vi "Generate Configuration.vi"(6 "Starting Address Offset":u16 format="%04x", 7 "Virtual Memory Unit in":refnum<class "Virtual Memory Unit.lvclass">, 8 "error in (no error)":errorcluster, 11 "Bus Controller in":refnum<class "Bus Controller.lvclass">) -> (0 "error out":errorcluster, 2 "Parameter List":string[](array[string]), 3 "Bus Controller out":refnum<class "Bus Controller.lvclass">, 4 "Next Address Offset":u16 format="%04x", 5 "Virtual Memory Unit out":refnum<class "Virtual Memory Unit.lvclass">)   [LabVIEW 2020, in "BCI-1553 API.lvlib" / "Bus Controller.lvclass"]
doc: "Generates the entire configuration for this Bus Controller. Does not push it to the Board component yet."
uses:
  Bus Controller.lvclass
  C:/Users/MattJ/Desktop/git/bci-1553-labview-api/src/1553 SubComponent/1553 SubComponent.lvclass
  Dependencies/Virtual Memory Unit/Virtual Memory Unit.lvclass
  Dependencies/Registry/Registry.lvclass/Registry.ctl
  Dependencies/Registry/Registry.lvclass
  1553 SubComponent/1553 SubComponent.lvclass
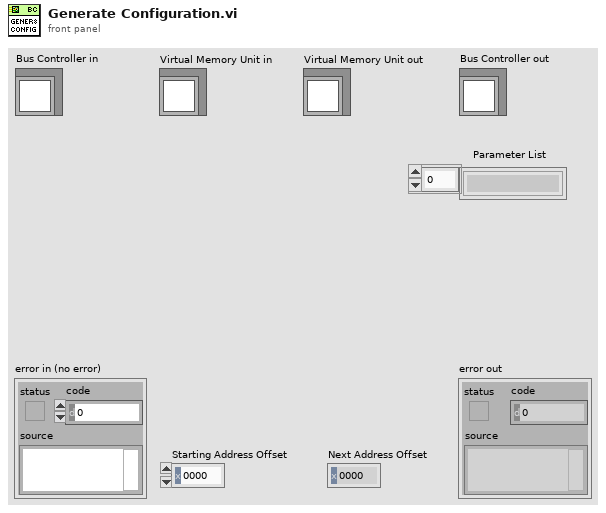
[diagram p1: front panel]
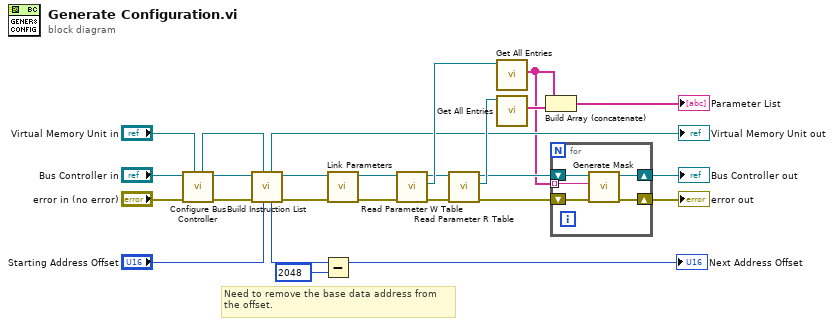
[diagram p0: block diagram]
diagram:
  # "Need to remove the base data address from\nthe offset."
  n1 = call "Configure Bus Controller.vi"("Virtual Memory Unit in"="Virtual Memory Unit in", "error in (no error)"="error in (no error)", "Bus Controller in"="Bus Controller in") -> ("error out"=w18:errorcluster, "Bus Controller out"=w21:refnum<class "Bus Controller.lvclass">, "Virtual Memory Unit out"=w14:refnum<class "Virtual Memory Unit.lvclass">)  [unwired: 6 in]
  n2 = call "Build Instruction List.vi"("Instruction List Starting Offset"="Starting Address Offset", "Virtual Memory Unit in"=w14, "error in (no error)"=w18, "Bus Controller in"=w21) -> ("error out"=w11:errorcluster, "Bus Controller out"=w12:refnum<class "Bus Controller.lvclass">, "Instruction List Final Address"=w3:u16, "Virtual Memory Unit out"=→"Virtual Memory Unit out":refnum<class "Virtual Memory Unit.lvclass">)  [unwired: 4 in]
  n3 = Subtract(x=w3, y=u16 2048) -> (x-y=→"Next Address Offset":u16)
  n4 = call "Link Parameters.vi"("error in (no error)"=w11, "Bus Controller in"=w12) -> ("error out"=w16:errorcluster, "Bus Controller out"=w19:refnum<class "Bus Controller.lvclass">)  [unwired: 8 in]
  n5 = call-dynamic "Read Parameter W Table.vi"("error in (no error)"=w16, "1553 SubComponent in"=w19) -> ("error out"=w26:errorcluster, "Parameter W Table"=w25:refnum<class "Registry.lvclass">, "1553 SubComponent out"=w23:refnum<class "Bus Controller.lvclass">)  [unwired: 7 in]
  n6 = call-dynamic "Read Parameter R Table.vi"("error in (no error)"=w26, "1553 SubComponent in"=w23) -> ("error out"=w8:errorcluster, "Parameter R Table"=w24:refnum<class "Registry.lvclass">, "1553 SubComponent out"=w9:refnum<class "Bus Controller.lvclass">)  [unwired: 7 in]
  n7 = call "Get All Entries.vi"("Registry in"=w25) -> ("Keys"=w5:string[])  [unwired: 8 in, 2 out]
  n8 = call "Get All Entries.vi"("Registry in"=w24) -> ("Keys"=w10:string[])  [unwired: 8 in, 2 out]
  n9 = Build Array (concatenate)(w5, w10) -> (→"Parameter List":string[])
  n10 = for {
    tunnel: w5 -> [w31] mode=indexing
    shift-right: [w29] -> w6
    shift-left: w9 -> [w30]
    shift-right: [w27] -> w7
    shift-left: w8 -> [w28]
    n11 = call "Generate Mask.vi"("error in (no error)"=w28, "Parameter"=w31, "1553 SubComponent in"=w30) -> ("error out"=w27:errorcluster, "1553 SubComponent out"=w29:refnum<class "Bus Controller.lvclass">)  [unwired: 7 in]
  }
  "error out" <- w7
  "Bus Controller out" <- w6
